vi "Configure Serial Bus (A429 - Basic).vi"(0 "VISA resource name":refnum<visa-resource-name>, 1 "Signal Type (2: Differential)":i32(ring)=2 items=["Line A", "Line B", "Differential"], 2 "Source (0: Channel 1)":i32(ring) items=["Channel 1", "Channel 2", "Channel 3", "Channel 4"], 5 "Serial Bus Name (1: Serial Bus 1)":i32(ring)=1 items=["Serial Bus 1"=1, "Serial Bus 2"=2], 7 "Display Base (1: Hex)":i32(ring)=1 items=["Binary", "Hex"], 9 "Word Decode Format (0: LDSDI)":i32(ring) items=["LDSDI", "LDSSM", "LDATA"], 11 "error in (no error)":errorcluster, 12 "Signal Speed (0: Low)":i32(ring) items=["Low", "High"]) -> (4 "VISA resource name out":refnum<visa-resource-name>, 15 "error out":errorcluster)   [LabVIEW 2016, in "Agilent 2000 3000 X-Series.lvlib"]
doc: "Configures the basic settings of ARINC 429 bus."
uses:
  Agilent 2000 3000 X-Series.lvlib
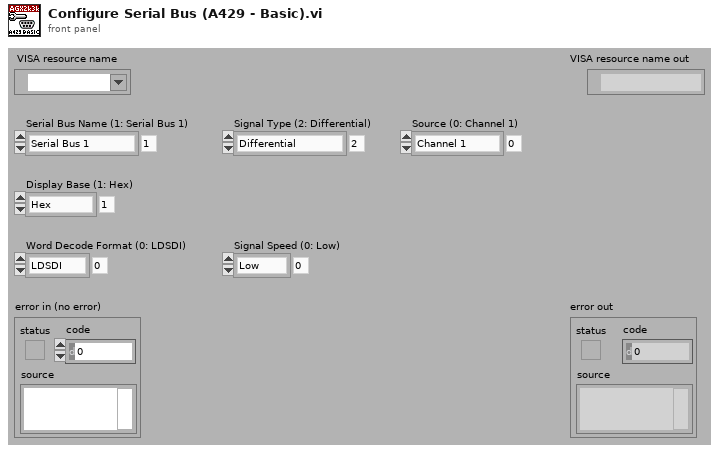
[diagram p1: front panel]
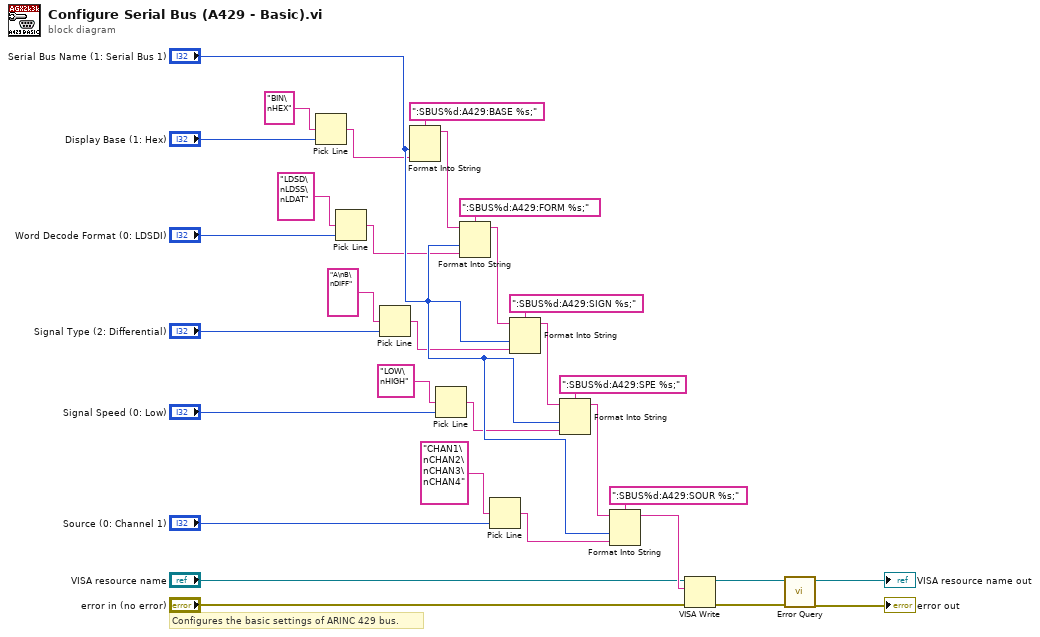
[diagram p0: block diagram]
diagram:
  # "Configures the basic settings of ARINC 429 bus."
  n1 = Pick Line(multi-line string="BIN\nHEX", line index="Display Base (1: Hex)") -> (output string=w28:string)  [unwired: 1 out]
  n2 = Pick Line(multi-line string="LDSD\nLDSS\nLDAT", line index="Word Decode Format (0: LDSDI)") -> (output string=w23:string)  [unwired: 1 out]
  n3 = Pick Line(multi-line string="A\nB\nDIFF", line index="Signal Type (2: Differential)") -> (output string=w18:string)  [unwired: 1 out]
  n4 = Format Into String(format string=":SBUS%d:A429:BASE %s;", "Serial Bus Name (1: Serial Bus 1)", w28) -> (resulting string=w25:string)  [unwired: 2 in, 1 out]
  n5 = Pick Line(multi-line string="LOW\nHIGH", line index="Signal Speed (0: Low)") -> (output string=w13:string)  [unwired: 1 out]
  n6 = Format Into String(format string=":SBUS%d:A429:FORM %s;", initial string=w25, "Serial Bus Name (1: Serial Bus 1)", w23) -> (resulting string=w20:string)  [unwired: 1 in, 1 out]
  n7 = Pick Line(multi-line string="CHAN1\nCHAN2\nCHAN3\nCHAN4", line index="Source (0: Channel 1)") -> (output string=w8:string)  [unwired: 1 out]
  n8 = Format Into String(format string=":SBUS%d:A429:SIGN %s;", initial string=w20, "Serial Bus Name (1: Serial Bus 1)", w18) -> (resulting string=w15:string)  [unwired: 1 in, 1 out]
  n9 = Format Into String(format string=":SBUS%d:A429:SPE %s;", initial string=w15, "Serial Bus Name (1: Serial Bus 1)", w13) -> (resulting string=w10:string)  [unwired: 1 in, 1 out]
  n10 = Format Into String(format string=":SBUS%d:A429:SOUR %s;", initial string=w10, "Serial Bus Name (1: Serial Bus 1)", w8) -> (resulting string=w7:string)  [unwired: 1 in, 1 out]
  n11 = VISA Write(VISA resource name="VISA resource name", write buffer=w7, error in (no error)="error in (no error)") -> (VISA resource name out=w4:refnum<visa-resource-name>, error out=w3:errorcluster)  [unwired: 1 out]
  n12 = call "Error Query.vi"("error in (no error)"=w3, "VISA resource name"=w4) -> ("error out"=→"error out":errorcluster, "VISA resource name out"=→"VISA resource name out":refnum<visa-resource-name>)  [unwired: 8 out]
